vi "Queue Nested Teardown.vi"(11 "jettl Queue Actor in":refnum<class "jettl Queue Actor.lvclass">) -> (3 "jettl Queue Actor out":refnum<class "jettl Queue Actor.lvclass">)   [LabVIEW 2021, in "jettl.lvlib" / "jettl Queue Actor.lvclass"]
uses:
  jettl Queue Actor.lvclass
  jettl Queue Actor.lvclass/jettl Queue Actor.ctl
  Actor/Msgs/Teardown/Teardown Msg/Teardown Msg.lvclass
  C:/git/jettl/src/Actor/Msgs/Teardown/Teardown Msg/Teardown Msg.lvclass
  C:/git/jettl/src/Actor/Msg/Msg.lvclass
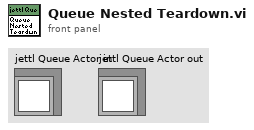
[diagram p1: front panel]
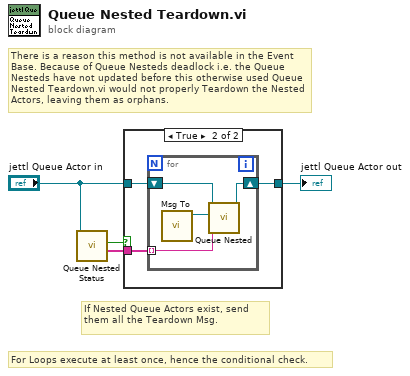
[diagram p0: block diagram]
diagram:
  # "For Loops execute at least once, hence the conditional check."
  # "If Nested Queue Actors exist, send them all the Teardown Msg."
  # "There is a reason this method is not available in the Event Base. Because of Queue Nesteds deadlock i.e. the Queue Nesteds have not updated before this otherwise used Queue Nested Teardown.vi would not properly Teardown the Nested Actors, leaving them as orphans."
  n1 = call-dynamic "Queue Nested Status.vi"("jettl Queue Actor in"="jettl Queue Actor in") -> ("Queue Nested Aliases"=w3:string[], "Any Exist?"=w4:bool)  [unwired: 8 in, 1 out]
  n2 = case shown="True" w4 {
    tunnel: [w5 w8] -> w1
    tunnel: "jettl Queue Actor in" -> [w5 w7]
    tunnel: w3 -> [_ w6]
    frame False {
    }
    frame True {
      n3 = for {
        tunnel: w6 -> [w11] mode=indexing
        shift-right: [w9] -> w8
        shift-left: w7 -> [w10]
        n4 = call "Msg To.vi"() -> ("Teardown Msg out"=w12:refnum<class "Teardown Msg.lvclass">)  [unwired: 11 in]
        n5 = call-dynamic "Queue Nested.vi"("Alias"=w11, "Msg"=w12, "jettl Queue Actor in"=w10) -> ("jettl Queue Actor out"=w9:refnum<class "jettl Queue Actor.lvclass">)  [unwired: 8 in]
      }
    }
  }
  "jettl Queue Actor out" <- w1
